vi "Start Asynchronous Calls to Array of Status Monitors.vi"(8 "error in":errorcluster, 10 "List of INI Files":path[](array[path]), 11 "New Status Received - Event Reference":refnum<user-event>) -> (0 "error out":errorcluster, 3 "References to Instances":refnum<vi>[](array[refnum]))   [LabVIEW 2017]
doc: "Starts a copy of the status monitor, for each unit under test that is defined by the list of INI files."
uses:
  Device Status and Index--Cluster.ctl
  Communications/Typedefs/DTACQ Module Carrier Status.ctl
  Communications/Typedefs/DTACQ Status--Enum.ctl
  Status Monitor/Status Monitor (Single Unit).vi
  Status Monitor/Status Monitor Library.lvlib
  Communications/Communications Library.lvlib
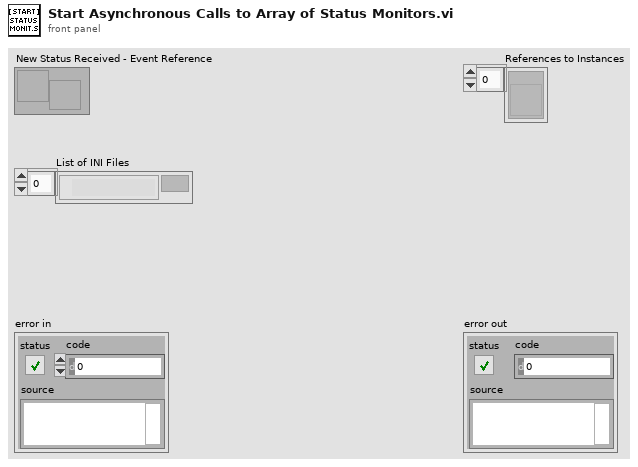
[diagram p1: front panel]
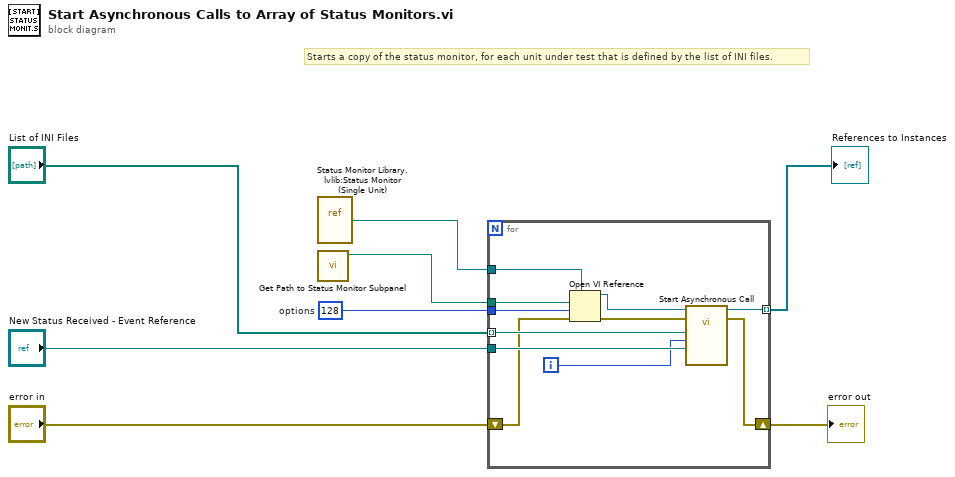
[diagram p0: block diagram]
diagram:
  w6 = 128  # options
  # "Starts a copy of the status monitor, for each unit under test that is defined by the list of INI files."
  n1 = vi-ref "Status Monitor Library.lvlib:Status Monitor (Single Unit).vi"() -> (w2:refnum<vi>)
  n2 = call "Get Path to Status Monitor Subpanel.vi"() -> ("Path to Status Monitor Subpanel"=w1:path)  [unwired: 11 in]
  n3 = for {
    tunnel: w1 -> [w19]
    tunnel: w2 -> [w18]
    tunnel: "List of INI Files" -> [w15] mode=indexing
    tunnel: "New Status Received - Event Reference" -> [w13]
    tunnel: [w14] -> w5 mode=indexing
    shift-right: [w11] -> w8
    shift-left: "error in" -> [w9]
    tunnel: w6 -> [w10]
    i -> [w12]
    n4 = Open VI Reference(type specifier VI Refnum (for type only)=w18, vi path=w19, options=w10, error in (no error)=w9) -> (vi reference=w17:refnum<vi>, error out=w16:errorcluster)  [unwired: 2 in]
    n5 = call-by-ref "Start Asynchronous Call"(reference=w17, error in=w16, "Update Status Event"=w13, "Device Index"=w12, "configuration file path"=w15) -> (reference out=w14:refnum<vi>, error out=w11:errorcluster)  [unwired: 9 in]
  }
  "error out" <- w8
  "References to Instances" <- w5
